vi "Build Node Graph Legend.vi"() -> (3 "Node Legend Graph":string)   [LabVIEW 2021, in "TAF Proj Document Type.lvlib" / "TAF Proj.lvclass"]
uses:
  <vilib>/Wovalab/AntiDoc/Document Type/Add-ons/LabVIEW TAF Project/TAF Proj/TAF Proj.lvclass
  <vilib>/Wovalab/AntiDoc/GraphBuilder/Renderer/Graphviz/Graphviz.lvclass
  C:/Program Files (x86)/National Instruments/LabVIEW 2021/vi.lib/Wovalab/AntiDoc/GraphBuilder/Renderer/Renderer.lvclass
  <vilib>/Wovalab/AntiDoc/GraphBuilder/Graph/Graph.lvclass
  <vilib>/Wovalab/AntiDoc/GraphBuilder/Shapes/Edge/Graphviz/Graphviz Edge Shape.lvclass
  <vilib>/Wovalab/AntiDoc/GraphBuilder/Shapes/Edge/Graphviz/Shape.ctl
  <vilib>/Wovalab/AntiDoc/GraphBuilder/Shapes/Edge/Graphviz/Colors.ctl
  <vilib>/Wovalab/AntiDoc/GraphBuilder/Shapes/Node/Graphviz/Colors.ctl
  <vilib>/Wovalab/AntiDoc/GraphBuilder/Shapes/Node/Graphviz/Shape.ctl
  <vilib>/Wovalab/AntiDoc/GraphBuilder/Node/Node.lvclass
  <vilib>/Wovalab/AntiDoc/GraphBuilder/Shapes/Node/Graphviz/Graphviz Node Shape.lvclass
  <vilib>/Wovalab/AntiDoc/GraphBuilder/Renderer/Graphviz/Graph Direction.ctl
  <vilib>/Wovalab/AntiDoc/GraphBuilder/Renderer/Graphviz/Specific Node Shape Def.ctl
  <vilib>/Wovalab/AntiDoc/Document Type/Add-ons/LabVIEW TAF Project/TAF Proj Document Type.lvlib
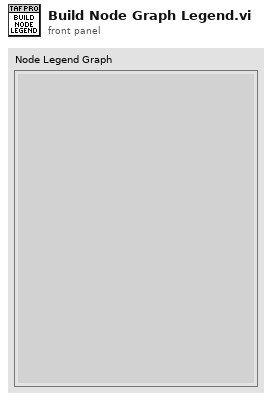
[diagram p1: front panel]
types:
  T1 = typedef "GraphBuilder.lvlib/Graphviz.lvclass/Specific Node Shape Def.ctl" = cluster{"Node ID":string, "Graphviz Node Shape":refnum<class "Graphviz Node Shape.lvclass">}
  T2 = typedef "GraphBuilder.lvlib/Graphviz.lvclass/Graph Direction.ctl" = enum16{"Top to Bottom", "Left To Right", "Bottom to Top", "Right to Left"}
  T3 = typedef "GraphBuilder.lvlib/Graphviz Node Shape.lvclass/Shape.ctl" = enum16{"box", "polygon", "ellipse", "oval", "circle", "point", "egg", "triangle", "plaintext", "plain", "diamond", "trapezium", "parallelogram", "house", "pentagon", "hexagon", "septagon", "octagon", "doublecircle", "doubleoctagon", "tripleoctagon", "invtriangle", "invtrapezium", "invhouse", "Mdiamond", "Msquare", "Mcircle", "rect", "rectangle", "square", "star", "none", "underline", "cylinder", "note", "tab", "folder", "box3D", "component", "promoter", "cds", "terminator", "utr", "primersite", "restrictionsite", "fivepoverhang", "threepoverhang", "noverhang", "assembly", "signature", "insulator", "ribosite", "rnastab", "proteasesite", "proteinstab", "rpromoter", "rarrow", "larrow", "lpromoter"}
  T4 = typedef "GraphBuilder.lvlib/Graphviz Node Shape.lvclass/Colors.ctl" = enum16{"aliceblue", "antiquewhite", "aqua", "aquamarine", "azure", "beige", "bisque", "black", "blanchedalmond", "blue", "blueviolet", "brown", "burlywood", "cadetblue", "chartreuse", "chocolate", "coral", "cornflowerblue", "cornsilk", "crimson", "cyan", "darkblue", "darkcyan", "darkgoldenrod", "darkgray", "darkgreen", "darkgrey", "darkkhaki", "darkmagenta", "darkolivegreen", "darkorange", "darkorchid", "darkred", "darksalmon", "darkseagreen", "darkslateblue", "darkslategray", "darkslategrey", "darkturquoise", "darkviolet", "deeppink", "deepskyblue", "dimgray", "dimgrey", "dodgerblue", "firebrick", "floralwhite", "forestgreen", "fuchsia", "gainsboro", "ghostwhite", "gold", "goldenrod", "gray", "green", "greenyellow", "grey", "honeydew", "hotpink", "indianred", "indigo", "ivory", "khaki", "lavender", "lavenderblush", "lawngreen", "lemonchiffon", "lightblue", "lightcoral", "lightcyan", "lightgoldenrodyellow", "lightgray", "lightgreen", "lightgrey", "lightpink", "lightsalmon", "lightseagreen", "lightskyblue", "lightslategray", "lightslategrey", "lightsteelblue", "lightyellow", "lime", "limegreen", "linen", "magenta", "maroon", "mediumaquamarine", "mediumblue", "mediumorchid", "mediumpurple", "mediumseagreen", "mediumslateblue", "mediumspringgreen", "mediumturquoise", "mediumvioletred", "midnightblue", "mintcream", "mistyrose", "moccasin", "navajowhite", "navy", "oldlace", "olive", "olivedrab", "orange", "orangered", "orchid", "palegoldenrod", "palegreen", "paleturquoise", "palevioletred", "papayawhip", "peachpuff", "peru", "pink", "plum", "powderblue", "purple", "red", "rosybrown", "royalblue", "saddlebrown", "salmon", "sandybrown", "seagreen", "seashell", "sienna", "silver", "skyblue", "slateblue", "slategray", "slategrey", "snow", "springgreen", "steelblue", "tan", "teal", "thistle", "tomato", "turquoise", "violet", "wheat", "white", "whitesmoke", "yellow", "yellowgreen"}
  T5 = typedef "GraphBuilder.lvlib/Graphviz Edge Shape.lvclass/Colors.ctl" = enum16{"aliceblue", "antiquewhite", "aqua", "aquamarine", "azure", "beige", "bisque", "black", "blanchedalmond", "blue", "blueviolet", "brown", "burlywood", "cadetblue", "chartreuse", "chocolate", "coral", "cornflowerblue", "cornsilk", "crimson", "cyan", "darkblue", "darkcyan", "darkgoldenrod", "darkgray", "darkgreen", "darkgrey", "darkkhaki", "darkmagenta", "darkolivegreen", "darkorange", "darkorchid", "darkred", "darksalmon", "darkseagreen", "darkslateblue", "darkslategray", "darkslategrey", "darkturquoise", "darkviolet", "deeppink", "deepskyblue", "dimgray", "dimgrey", "dodgerblue", "firebrick", "floralwhite", "forestgreen", "fuchsia", "gainsboro", "ghostwhite", "gold", "goldenrod", "gray", "green", "greenyellow", "grey", "honeydew", "hotpink", "indianred", "indigo", "ivory", "khaki", "lavender", "lavenderblush", "lawngreen", "lemonchiffon", "lightblue", "lightcoral", "lightcyan", "lightgoldenrodyellow", "lightgray", "lightgreen", "lightgrey", "lightpink", "lightsalmon", "lightseagreen", "lightskyblue", "lightslategray", "lightslategrey", "lightsteelblue", "lightyellow", "lime", "limegreen", "linen", "magenta", "maroon", "mediumaquamarine", "mediumblue", "mediumorchid", "mediumpurple", "mediumseagreen", "mediumslateblue", "mediumspringgreen", "mediumturquoise", "mediumvioletred", "midnightblue", "mintcream", "mistyrose", "moccasin", "navajowhite", "navy", "oldlace", "olive", "olivedrab", "orange", "orangered", "orchid", "palegoldenrod", "palegreen", "paleturquoise", "palevioletred", "papayawhip", "peachpuff", "peru", "pink", "plum", "powderblue", "purple", "red", "rosybrown", "royalblue", "saddlebrown", "salmon", "sandybrown", "seagreen", "seashell", "sienna", "silver", "skyblue", "slateblue", "slategray", "slategrey", "snow", "springgreen", "steelblue", "tan", "teal", "thistle", "tomato", "turquoise", "violet", "wheat", "white", "whitesmoke", "yellow", "yellowgreen"}
  T6 = typedef "GraphBuilder.lvlib/Graphviz Edge Shape.lvclass/Shape.ctl" = enum16{"box", "lbox", "rbox", "obox", "olbox", "orbox", "crow", "lcrow", "rcrow", "diamond", "ldiamond", "rdiamond", "odiamond", "oldiamond", "ordiamond", "dot", "odot", "inv", "linv", "rinv", "oinv", "olinv", "orinv", "none", "normal", "lnormal", "rnormal", "onormal", "olnormal", "ornormal", "tee", "ltee", "rtee", "vee", "lvee", "rvee", "curve", "lcurve", "rcurve", "icurve", "licurve", "ricurve"}
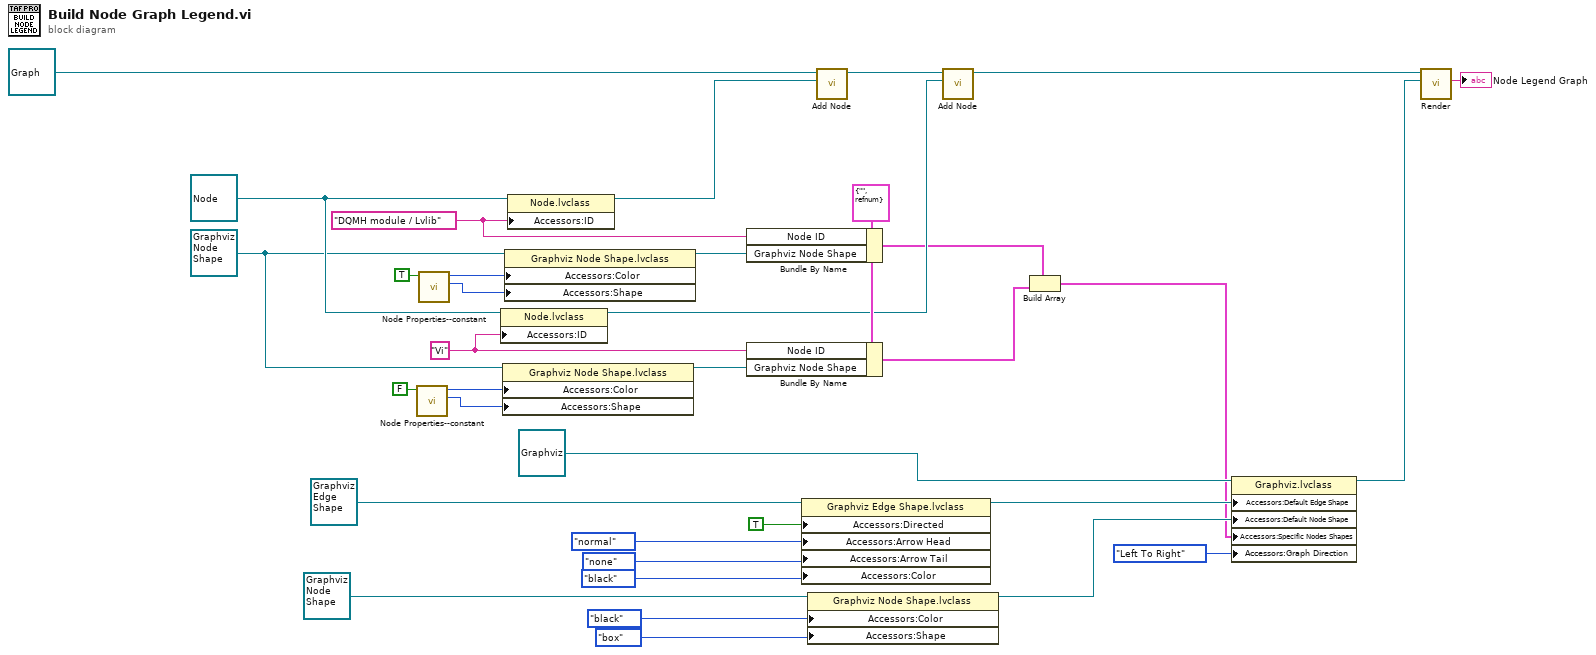
[diagram p0: block diagram]
diagram:
  w14 = T1 {"Node ID"="", "Graphviz Node Shape"=refnum} ("Specific Node Shape")
  w10 = "Vi" ("ID")
  w11 = "DQMH module / Lvlib" ("ID")
  w7 = refnum<class "Graphviz Node Shape.lvclass"> refnum ("GraphBuilder.lvlib:Graphviz Node Shape.lvclass")
  w8 = refnum<class "Node.lvclass"> refnum ("GraphBuilder.lvlib:Node.lvclass")
  n1 = call <vilib>:"Node Properties--constant.vi"("Lvlib"=FALSE) -> ("Shape"=w20:T3, "Color"=w9:T4)  [unwired: 9 in]
  n2 = call <vilib>:"Node Properties--constant.vi"("Lvlib"=TRUE) -> ("Shape"=w17:T3, "Color"=w18:T4)  [unwired: 9 in]
  n3 = property class="Node.lvclass"(reference=w8, "Accessors:ID"=w10) -> (reference out=w13:refnum<class "Node.lvclass">)  [unwired: 1 in, 1 out]
  n4 = property class="Graphviz Node Shape.lvclass"(reference=w7, "Accessors:Color"=w9, "Accessors:Shape"=w20) -> (reference out=w23:refnum<class "Graphviz Node Shape.lvclass">)  [unwired: 1 in, 1 out]
  n5 = property class="Graphviz Node Shape.lvclass"(reference=w7, "Accessors:Color"=w18, "Accessors:Shape"=w17) -> (reference out=w15:refnum<class "Graphviz Node Shape.lvclass">)  [unwired: 1 in, 1 out]
  n6 = property class="Node.lvclass"(reference=w8, "Accessors:ID"=w11) -> (reference out=w19:refnum<class "Node.lvclass">)  [unwired: 1 in, 1 out]
  n7 = Bundle By Name(cluster=w14, "Node ID"=w11, "Graphviz Node Shape"=w15) -> (w3:T1)
  n8 = Bundle By Name(cluster=w14, "Node ID"=w10, "Graphviz Node Shape"=w23) -> (w2:T1)
  n9 = property class="Graphviz Edge Shape.lvclass"(reference=refnum<class "Graphviz Edge Shape.lvclass"> refnum ("GraphBuilder.lvlib:Graphviz Edge Shape.lvclass"), "Accessors:Directed"=TRUE ("Directed"), "Accessors:Arrow Head"=Shape."normal" ("Arrow Head"), "Accessors:Arrow Tail"=Shape."none" ("Arrow Tail"), "Accessors:Color"=Colors."black" ("Color")) -> (reference out=w33:refnum<class "Graphviz Edge Shape.lvclass">)  [unwired: 1 in, 1 out]
  n10 = property class="Graphviz Node Shape.lvclass"(reference=refnum<class "Graphviz Node Shape.lvclass"> refnum ("GraphBuilder.lvlib:Graphviz Node Shape.lvclass"), "Accessors:Color"=Colors."black" ("Color"), "Accessors:Shape"=Shape."box" ("Shape")) -> (reference out=w34:refnum<class "Graphviz Node Shape.lvclass">)  [unwired: 1 in, 1 out]
  n11 = call-dynamic "Add Node.vi"("Node"=w19, "Graph in"=refnum<class "Graph.lvclass"> refnum ("GraphBuilder.lvlib:Graph.lvclass")) -> ("Graph out"=w5:refnum<class "Graph.lvclass">)  [unwired: 8 in, 1 out]
  n12 = call-dynamic "Add Node.vi"("Node"=w13, "Graph in"=w5) -> ("Graph out"=w4:refnum<class "Graph.lvclass">)  [unwired: 8 in, 1 out]
  n13 = Build Array(w3, w2) -> (w1:T1[])
  n14 = property class="Graphviz.lvclass"(reference=refnum<class "Graphviz.lvclass"> refnum ("GraphBuilder.lvlib:Graphviz.lvclass"), "Accessors:Default Edge Shape"=w33, "Accessors:Default Node Shape"=w34, "Accessors:Specific Nodes Shapes"=w1, "Accessors:Graph Direction"=Graph_Direction."Left To Right" ("Graph Direction")) -> (reference out=w35:refnum<class "Graphviz.lvclass">)  [unwired: 1 in, 1 out]
  n15 = call-dynamic "Render.vi"("Renderer"=w35, "Graph in"=w4) -> ("Rendered Stream"=→"Node Legend Graph":string)  [unwired: 7 in, 2 out]
